vi "DispenseMarble.vi"(1 "Input":T1) -> (0 "Output":T1)   [LabVIEW 2016]
uses:
  <vilib>/NXT/Subs/LVHSConnector.ctl
  <vilib>/NXT/LegoClasses/BrickReference/BrickReference.lvclass
  <vilib>/NXT/Block Support/NXT_OutputPort.ctl
  <vilib>/NXT/NXTIO Xnodes/NXTIONodeSubVIs/NXTMotorRunDistance.vi
  <vilib>/NXT/Dual Mode Library/Waits/Wait_Num.vi
  <vilib>/NXT/NXTIO Xnodes/AddressXNode/NXTIOAddress.xnode
  <vilib>/NXT/NXTIO Xnodes/NXTIOXNode/NXTIO.xnode
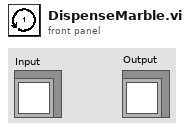
[diagram p1: front panel]
types:
  T1 = typedef "LVHSConnector.ctl" = refnum<class "BrickReference.lvclass">
  T2 = typedef "NXT_OutputPort.ctl" = u8
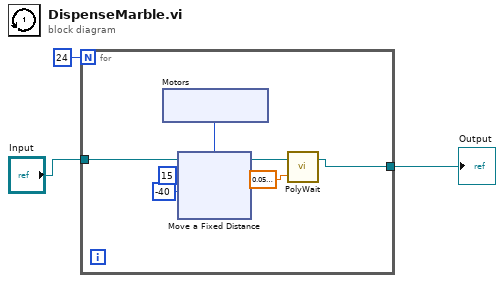
[diagram p0: block diagram]
diagram:
  n1 = for {
    N: 24 -> [_]
    tunnel: [w5] -> w2
    tunnel: "Input" -> [w4]
    n2 = xnode "Motors"() -> ("Motor"=w6:T2)
    n3 = xnode "Move a Fixed Distance"("Speed 1"=i8 -40, "Distance 1"=15, "Motors"=w6, "NXT/EV3"=w4) -> ("NXT/EV3"=w10:T1)
    n4 = call-poly <vilib>:"PolyWait.vi"("Time (1 sec)"=sgl 0.05, "NXT/EV3"=w10) -> ("NXT/EV3"=w5:T1)  [unwired: 2 in]
  }
  "Output" <- w2
